vi "手动配置经纬度.vi"(10 "经度输入":dbl, 11 "纬度输入":dbl) -> (2 "经度":dbl, 3 "纬度":dbl)   [LabVIEW 2016, in "环境动力监测库.lvlib" / "NMEA.lvlib"]
uses:
  NMEA.lvlib
panel:
  in  "取消":bool
  in  "确定":bool
  # "设置经纬度信息"
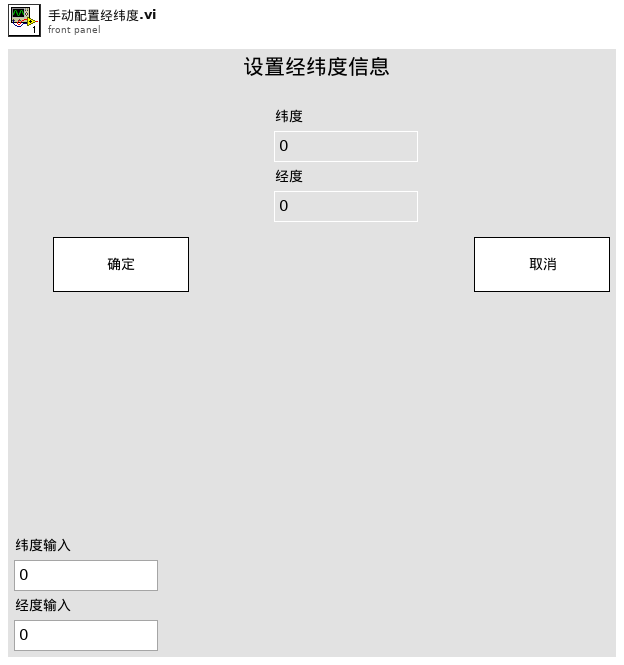
[diagram p1: front panel]
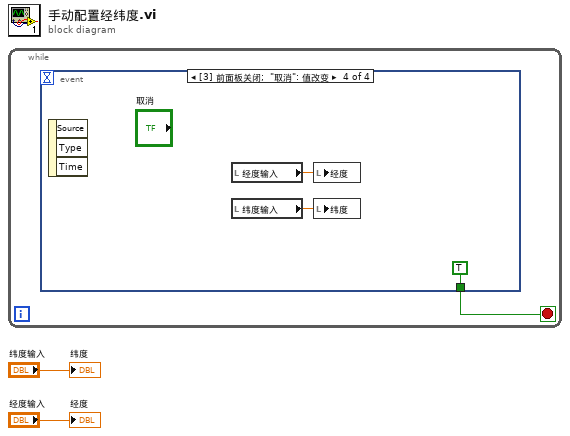
[diagram p0: block diagram]
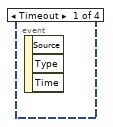
[diagram p2: hidden frame]
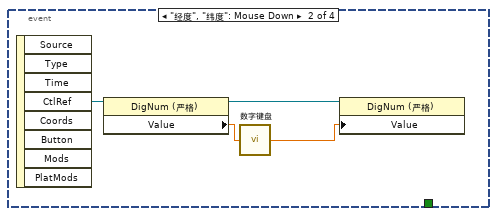
[diagram p3: hidden frame]
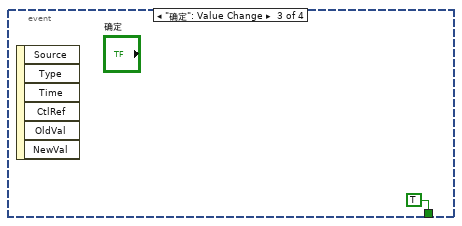
[diagram p4: hidden frame]
diagram:
  n1 = while {
    stop <- w3 stop-if-true
    n2 = event shown="[3] 前面板关闭;  \"取消\": 值改变" {
      selector: _ -> [_ _ _ _]
      dyn-events: _ -> [_ _ _ _]
      timeout: _ -> [_ _ _ _]
      tunnel: [_ _ TRUE TRUE] -> w3
      event Timeout {
        n3 = event-data() -> ()  [unwired: 1 in, 3 out]
      }
      event "经度", "纬度": Mouse Down {
        n4 = event-data() -> ("CtlRef"=w7:refnum<vi>)  [unwired: 1 in, 7 out]
        n5 = property class="DigNum (严格)"(reference=w7) -> (reference out=w5:refnum<vi>, "Value"=w6:dbl)  [unwired: 1 in, 1 out]
        n6 = call "数字键盘.vi"("OldNumber"=w6) -> ("NewNumber"=w4:dbl)
        n7 = property class="DigNum (严格)"(reference=w5, "Value"=w4) -> ()  [unwired: 1 in, 2 out]
      }
      event "确定": Value Change {
        n8 = event-data() -> ()  [unwired: 1 in, 6 out]
      }
      event Panel Close; "取消": Value Change {
        n9 = event-data() -> ()  [unwired: 1 in, 3 out]
        n10 = local read "经度输入"() -> (w10:dbl)
        n11 = local read "纬度输入"() -> (w11:dbl)
        n12 = local write "经度"(w10) -> ()
        n13 = local write "纬度"(w11) -> ()
      }
    }
  }
  "经度" <- "经度输入"
  "纬度" <- "纬度输入"
